vi "NT Read Value.vi"   [LabVIEW 2017]
doc: "A polyVI that will return the data of the named entry. Use the poly selector to choose the type to read."
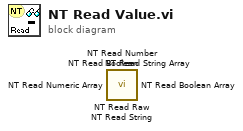
[diagram p0: block diagram]
diagram:
  n1 = call <vilib>:"NT Read Raw.vi"() -> ()  [unwired: 10 in, 2 out]
  n2 = call <vilib>:"NT Read String Array.vi"() -> ()  [unwired: 10 in, 2 out]
  n3 = call <vilib>:"NT Read Numeric Array.vi"() -> ()  [unwired: 10 in, 2 out]
  n4 = call <vilib>:"NT Read Boolean Array.vi"() -> ()  [unwired: 10 in, 2 out]
  n5 = call <vilib>:"NT Read String.vi"() -> ()  [unwired: 10 in, 2 out]
  n6 = call <vilib>:"NT Read Number.vi"() -> ()  [unwired: 10 in, 2 out]
  n7 = call <vilib>:"NT Read Boolean.vi"() -> ()  [unwired: 10 in, 2 out]
